vi "ToTable.vi"(8 "error in (no error)":errorcluster, 10 "variant":variant, 11 "node in":refnum<class "Table Test Editor Node.lvclass">) -> (0 "error out":errorcluster, 2 "table":string[][](array[string]), 3 "node in out":refnum<class "Table Test Editor Node.lvclass">)   [LabVIEW 2013, in "Table Test Editor Node.lvclass"]
doc: "Copyright 2015 National Instruments Corporation\n\nLicensed under the Apache License, Version 2.0 (the \"License\"); you may not use this file except in compliance with the License. You may obtain a copy of the License at http://www.apache.org/licenses/LICENSE-2.0\nUnless required by applicable law or agreed to in writing, software distributed under the License is distributed on an \"AS IS\" BASIS, WITHOUT WARRANTIES OR CONDITIONS OF ANY KIND, either express or implied. See the License for the specific language governing permissions and limitations under the License."
uses:
  Table Test Editor Node.lvclass
  <vilib>/NI/Tag Bus/tag/tag descriptor.lvclass
  <vilib>/NI/Module Execution Interface/Engine Configuration/engine configuration.lvclass
  Table Test Editor Node.lvclass/Table Test Editor Node.ctl
  module/configuration/Table Test configuration.lvclass/Table Test configuration.ctl
  <vilib>/NI/Configuration Framework/serializable configuration/NISE_CEF_serializable configuration.lvclass/NISE_CEF_serializable configuration.ctl
  <vilib>/NI/Module Execution Interface/Engine Configuration/engine configuration.lvclass/engine configuration.ctl
  <vilib>/NI/Tag Bus/tag/tag descriptor.lvclass/tag descriptor.ctl
  module/configuration/Read tag select.vi
  <vilib>/Utility/LVClass/Get LV Class Name.vi
  <vilib>/NI/Configuration Framework/error generator/NISE_error generator.vi
  <vilib>/NI/Configuration Framework/serializable configuration/NISE_CEF_serializable configuration.lvclass
  module/configuration/Table Test configuration.lvclass
panel:
  out "tag list":refnum<class "tag descriptor.lvclass">[](array[class])
  out "error out 2":errorcluster
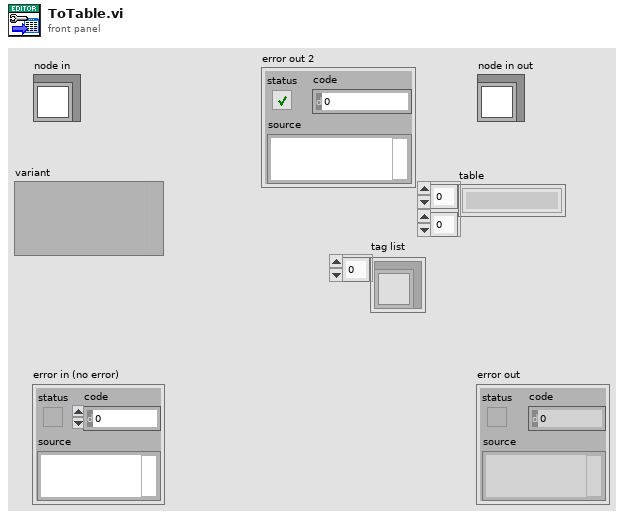
[diagram p1: front panel]
types:
  T1 = typedef "tag select module configuration.lvclass/tag select configuration.ctl" = cluster{"tag select name":string, "data type":T2, "output":refnum<class "TBM channel.lvclass">, "select":refnum<class "TBM channel.lvclass">, "input channels":refnum<class "TBM channel.lvclass">[]}
  T2 = typedef "tag bus.lvlib/tag descriptor.lvclass/Data Type.ctl" = enum16{"Double", "Single", "I64", "I32", "I16", "I8", "U64", "U32", "U16", "U8", "Boolean", "String", "Array of Double", "Array of Single", "Array of I64", "Array of I32", "Array of I16", "Array of I8", "Array of U64", "Array of U32", "Array of U16", "Array of U8", "Array of Boolean", "Array of String"}
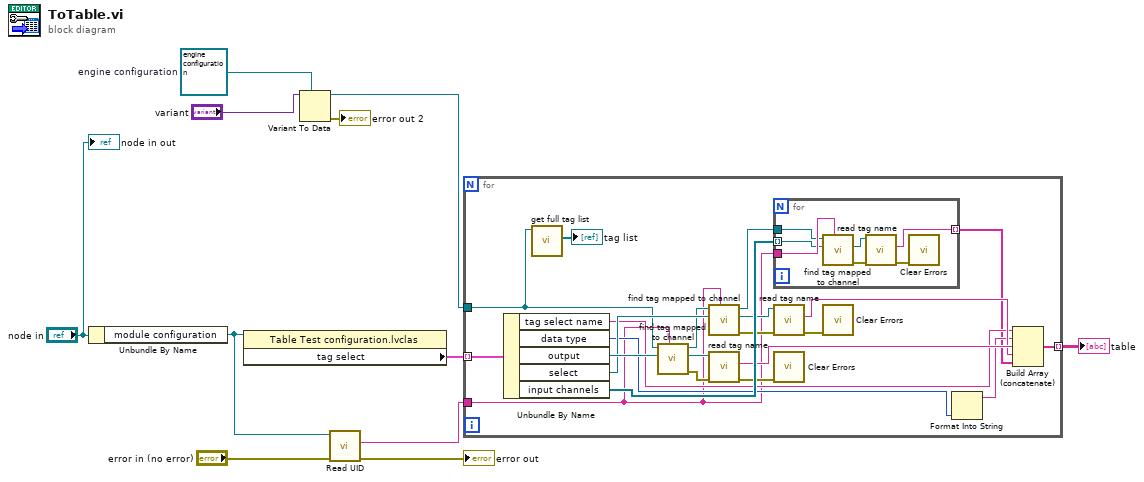
[diagram p0: block diagram]
diagram:
  w8 = refnum<class "engine configuration.lvclass"> refnum  # engine configuration
  n1 = Unbundle By Name("node in") -> ("module configuration"=w3:refnum<class "Table Test configuration.lvclass">)
  n2 = property class="Table Test configuration.lvclas"(reference=w3) -> ("tag select"=w10:T1[])  [unwired: 1 in, 2 out]
  n3 = Variant To Data(type=w8, Variant="variant") -> (data=w9:refnum<class "engine configuration.lvclass">, error out=→"error out 2":errorcluster)  [unwired: 1 in]
  n4 = call <vilib>:"Read UID.vi"("error in"="error in (no error)", "configuration in"=w3) -> ("error out"=→"error out":errorcluster, "instance id"=w11:string)  [unwired: 7 in, 1 out]
  n5 = for {
    tunnel: w10 -> [w33] mode=indexing
    tunnel: w9 -> [w13]
    tunnel: w11 -> [w14]
    tunnel: [w21] -> w7 mode=indexing
    n6 = Unbundle By Name(w33) -> ("tag select name"=w25:string, "data type"=w24:T2, "output"=w30:refnum<class "TBM channel.lvclass">, "select"=w29:refnum<class "TBM channel.lvclass">, "input channels"=w31:refnum<class "TBM channel.lvclass">[])
    n7 = call <vilib>:"get full tag list.vi"("engine configuration in"=w13) -> ("tag list"=→"tag list":refnum<class "tag descriptor.lvclass">[])  [unwired: 9 in, 1 out]
    n8 = call <vilib>:"find tag mapped to channel.vi"("owner"=w14, "channel"=w30, "engine configuration in"=w13) -> ("error out"=w18:errorcluster, "tag"=w32:refnum<class "tag descriptor.lvclass">, "engine configuration out"=w19:refnum<class "engine configuration.lvclass">)  [unwired: 6 in]
    n9 = call <vilib>:"find tag mapped to channel.vi"("owner"=w14, "channel"=w29, "engine configuration in"=w19) -> ("error out"=w17:errorcluster, "tag"=w27:refnum<class "tag descriptor.lvclass">, "engine configuration out"=w20:refnum<class "engine configuration.lvclass">)  [unwired: 6 in]
    n10 = call <vilib>:"read tag name.vi"("error in"=w18, "system tag in"=w32) -> ("error out"=w15:errorcluster, "name"=w28:string)  [unwired: 7 in, 1 out]
    n11 = for {
      tunnel: w14 -> [w40]
      tunnel: w31 -> [w39] mode=indexing
      tunnel: [w37] -> w22 mode=indexing
      tunnel: w20 -> [w36]
      n12 = call <vilib>:"find tag mapped to channel.vi"("owner"=w40, "channel"=w39, "engine configuration in"=w36) -> ("error out"=w35:errorcluster, "tag"=w38:refnum<class "tag descriptor.lvclass">)  [unwired: 6 in, 1 out]
      n13 = call <vilib>:"read tag name.vi"("error in"=w35, "system tag in"=w38) -> ("error out"=w34:errorcluster, "name"=w37:string)  [unwired: 7 in, 1 out]
      n14 = call <vilib>:"Clear Errors.vi"("error in (no error)"=w34) -> ()  [unwired: 6 in, 1 out]
    }
    n15 = call <vilib>:"read tag name.vi"("error in"=w17, "system tag in"=w27) -> ("error out"=w16:errorcluster, "name"=w26:string)  [unwired: 7 in, 1 out]
    n16 = call <vilib>:"Clear Errors.vi"("error in (no error)"=w15) -> ()  [unwired: 6 in, 1 out]
    n17 = call <vilib>:"Clear Errors.vi"("error in (no error)"=w16) -> ()  [unwired: 6 in, 1 out]
    n18 = Format Into String(w24) -> (resulting string=w23:string)  [unwired: 3 in, 1 out]
    n19 = Build Array (concatenate)(w25, w23, w28, w26, w22) -> (w21:string[])
  }
  "table" <- w7
  "node in out" <- "node in"
